vi "DB SQL Select.vi"(8 "error in (no error)":errorcluster, 10 "Table Name":string="Contacts", 11 "Connection Information":path=path "MySQL.dsn") -> (0 "error out":errorcluster, 3 "Data":string[][](table))   [LabVIEW 2011]
doc: "Executes a SELECT * query on the database and table passed in.\n\n<b>Connection Information</b> - Path to the file DSN for connection to the ODBC database.\n\n<b>Table Name</b> - Name of the table in the database to perform the SELECT * query.\n\n\nVersion 1.0 - 10/20/2009\n\nPhaeron, Inc.\nwww.phaeron.com\ninfo@phaeron.com"
uses:
  <vilib>/addons/database/NI_Database_API.lvlib
  <vilib>/addons/database/Connection.llb/DB Tools Open Connec (Path).vi
  <vilib>/addons/database/_DB Variant To Data/Database Variant To Data.xnode
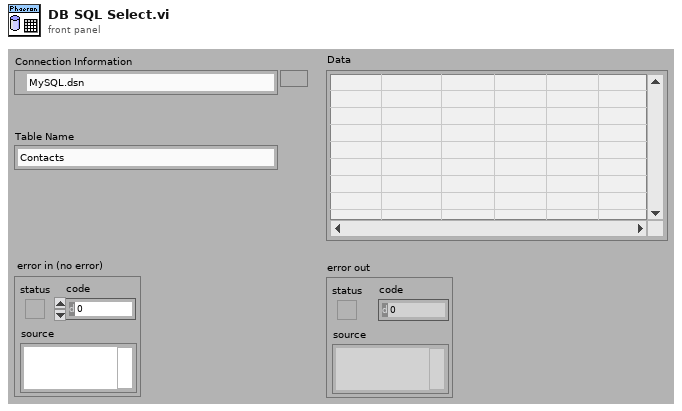
[diagram p1: front panel]
types:
  T1 = typedef "NI_Database_API.lvlib/Conn ObjectReference.ctl" = refnum<k1>
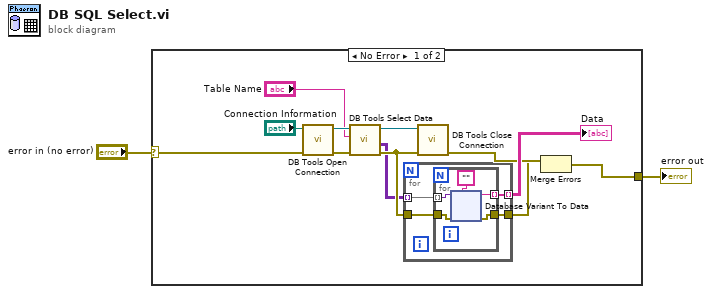
[diagram p0: block diagram]
diagram:
  n1 = case shown="No Error" "error in (no error)" {
    selector: "error in (no error)" -> [w4 w56]
    tunnel: [w5 w56] -> w2
    frame No Error {
      n2 = call-poly <vilib>:"DB Tools Open Connection.vi"("error in (no error)"=w4, "connection information"="Connection Information") -> ("error out"=w11:errorcluster, "connection reference"=w13:T1)  [unwired: 6 in]
      n3 = call <vilib>:"DB Tools Select Data.vi"("error in (no error)"=w11, "table"="Table Name", "connection reference"=w13) -> ("error out"=w8:errorcluster, "data"=w3:variant[][], "connection reference out"=w12:T1)  [unwired: 3 in]
      n4 = for {
        tunnel: [w18] -> w9 mode=indexing
        tunnel: w3 -> [w17] mode=indexing
        tunnel: w8 -> [w16]
        tunnel: [w15] -> w6
        n5 = for {
          tunnel: [w22] -> w18 mode=indexing
          tunnel: w17 -> [w21] mode=indexing
          tunnel: w16 -> [w20]
          tunnel: [w19] -> w15
          n6 = xnode "Database Variant To Data"("database variant"=w21, "error in"=w20, "type"="") -> ("data"=w22:string, "error out"=w19:errorcluster)
        }
      }
      "Data" <- w9
      n7 = call <vilib>:"DB Tools Close Connection.vi"("error in (no error)"=w8, "connection reference"=w12) -> ("error out"=w7:errorcluster)  [unwired: 5 in]
      n8 = Merge Errors(w7, w6) -> (w5:errorcluster)
    }
    frame Error {
    }
  }
  "error out" <- w2
